vi "getLaserStatus.vi"(8 "error in (no error)":errorcluster, 11 "Monochromator in":refnum<class "Monochromator.lvclass">) -> (0 "error out":errorcluster, 3 "Monochromator out":refnum<class "Monochromator.lvclass">)   [LabVIEW 2023, in "Monochromator.lvclass"]
uses:
  Monochromator.lvclass
  d9b87029-586e-44ee-a6e5-d4a5e0edce38.vi
  b59fd1e7-dcda-425c-bd6c-61aafb79e7f4.vi
  GenericDevice/GenericDevice.lvclass
  <vilib>/IlluminatedG/lv-web-crypto/lv-json/JSON/JSON.lvlib
panel:
  # "Connector Pane"
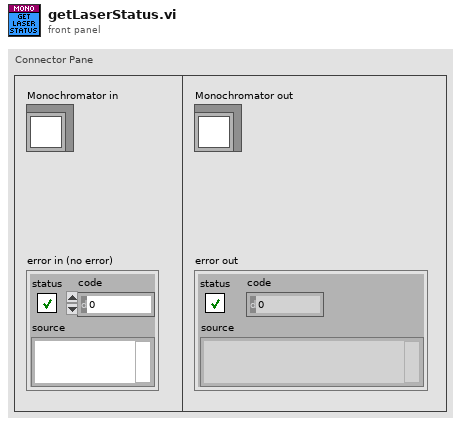
[diagram p1: front panel]
types:
  T1 = typedef "Monochromator.lvclass/ShutterStatus.ctl" = cluster{"Shutter 1":i32, "Shutter 2":i32}
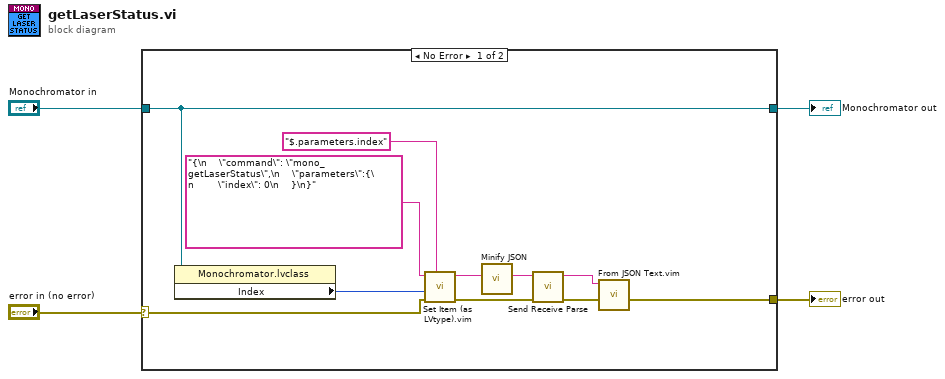
[diagram p0: block diagram]
diagram:
  n1 = case shown="No Error" "error in (no error)" {
    selector: "error in (no error)" -> [w13 w19]
    tunnel: [w12 w19] -> w3
    tunnel: [w15 w18] -> w1
    tunnel: "Monochromator in" -> [w15 w18]
    frame No Error {
      n2 = property class="Monochromator.lvclass"(reference=w15) -> ("Index"=w14:i32)  [unwired: 1 in, 2 out]
      n3 = call "Set Item (as LVtype).vim"("$Path or Item Name"="$.parameters.index", "error in (no error)"=w13, "Anything"=w14, "JSON"="{\n    \"command\": \"mono_getLaserStatus\",\n    \"parameters\":{\n        \"index\": 0\n    }\n}") -> ("error out"=w11:errorcluster, "<JSON>"=w8:string)  [unwired: 4 in, 1 out]
      n4 = call <vilib>:"Minify JSON.vi"("JSON String"=w8) -> ("Minified JSON"=w7:string)  [unwired: 10 in]
      n5 = call "Send Receive Parse.vi"("error in"=w11, "<JSON>"=w7) -> ("error out"=w9:errorcluster, "results-JSON string"=w10:string)  [unwired: 7 in, 1 out]
      n6 = call "From JSON Text.vim"("error in (no error)"=w9, "JSON"=w10) -> ("error out"=w12:errorcluster, "Data out"=w6:T1, "Data Type and Default Value"=w5:T1)  [unwired: 7 in]
    }
    frame Error {
    }
  }
  "error out" <- w3
  "Monochromator out" <- w1
